vi "XYZ_XYStage_Status.vi"(4 "Model":string, 5 "error in (no error)":errorcluster, 7 "nStatusTries":i32=100, 8 "VISA resource name":refnum<visa-resource-name>="COM1") -> (0 "error out":errorcluster, 2 "Successs":bool, 3 "VISA resource name out":refnum<visa-resource-name>="COM1")   [LabVIEW 2013]
doc: "Sends STATUS command every 50 ms up to nStatusTries times.\nIf reply 'N' is received within nStatusTries times, then returns with Success = TRUE,\nelse returns with Success = FALSE."
uses:
  <vilib>/Instr/_visa.llb/VISA Configure Serial Port (Instr).vi
  Global.vi
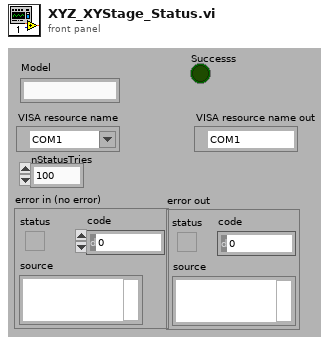
[diagram p1: front panel]
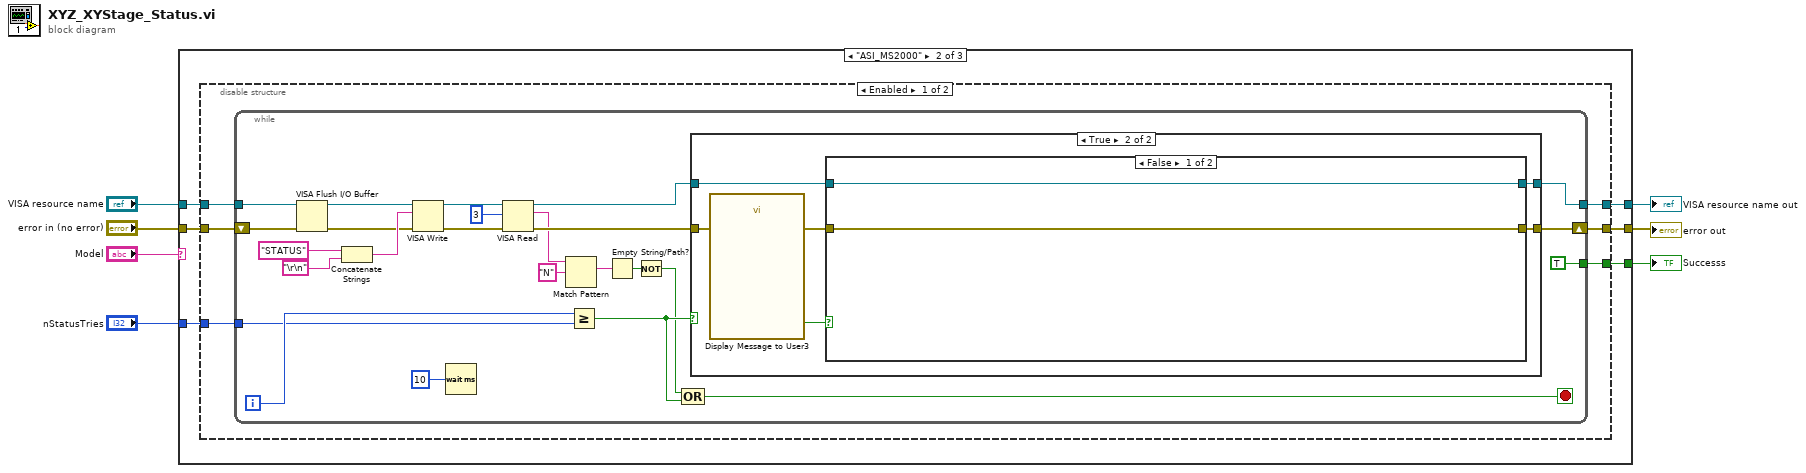
[diagram p0: block diagram]
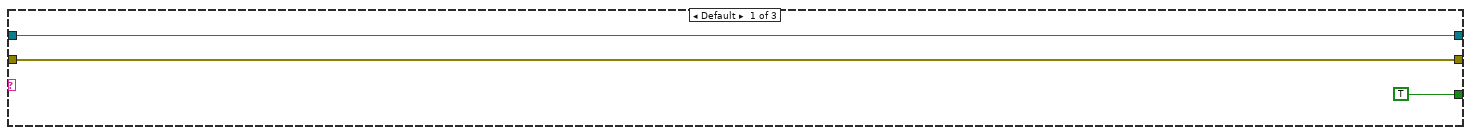
[diagram p2: hidden frame]
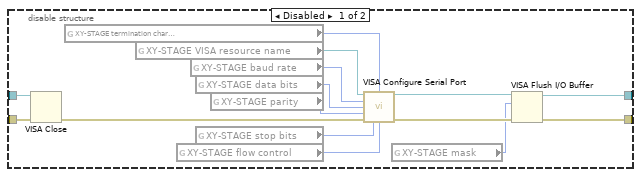
[diagram p5: hidden frame]
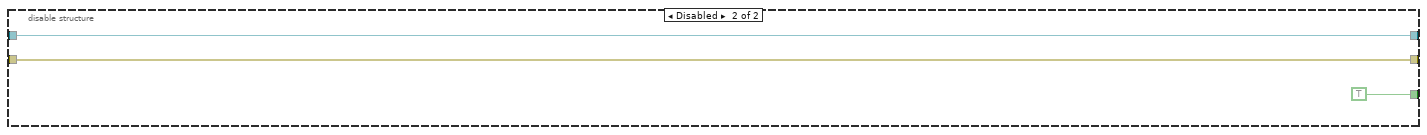
[diagram p6: hidden frame]
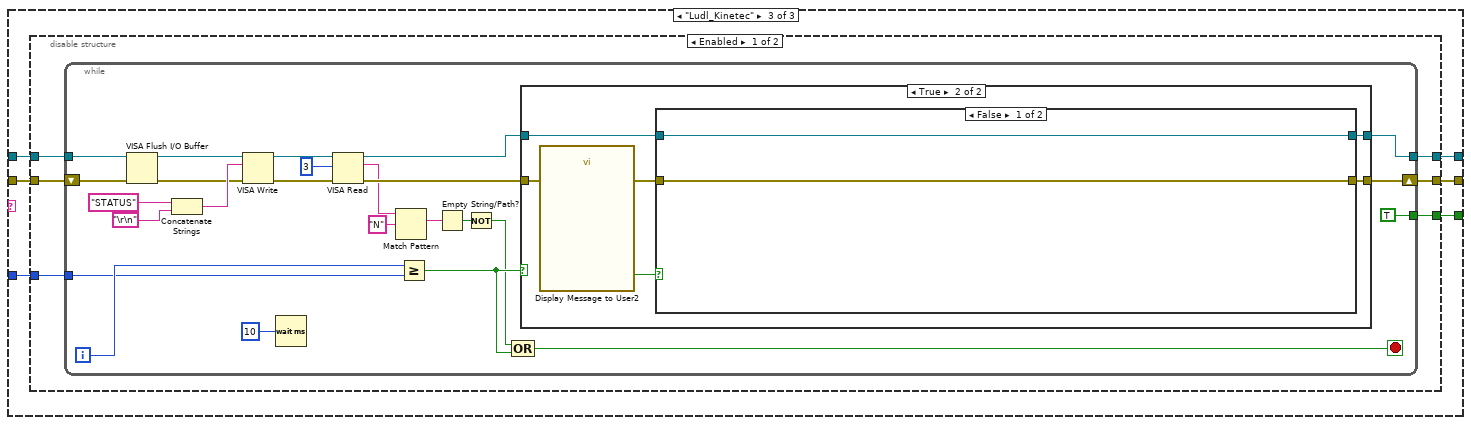
[diagram p7: hidden frame]
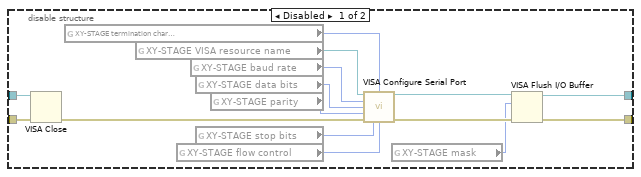
[diagram p10: hidden frame]
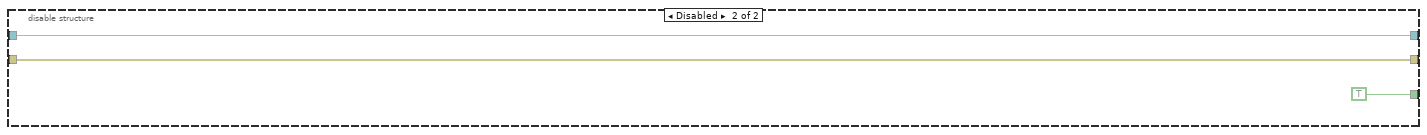
[diagram p11: hidden frame]
diagram:
  n1 = case shown="\"ASI_MS2000\"" "Model" {
    tunnel: [w9 w13 w84] -> w7
    tunnel: "error in (no error)" -> [w9 w16 w87]
    tunnel: "VISA resource name" -> [w8 w15 w86]
    tunnel: [TRUE w14 w85] -> w4
    tunnel: "nStatusTries" -> [_ w12 w83]
    tunnel: [w8 w11 w82] -> w1
    frame Default {
    }
    frame "ASI_MS2000" {
      n2 = disable-structure shown="Enabled" {
        disable-tunnel: w16 -> [w22 w81]
        disable-tunnel: w15 -> [w21 w79]
        disable-tunnel: [w20 TRUE] -> w14
        disable-tunnel: [w19 w81] -> w13
        disable-tunnel: w12 -> [w18 _]
        disable-tunnel: [w17 w79] -> w11
        frame Enabled {
          n3 = while {
            tunnel: w21 -> [w46]
            tunnel: [TRUE] -> w20
            shift-right: [w42] -> w19
            shift-left: w22 -> [w45]
            tunnel: w18 -> [w41]
            tunnel: [w28] -> w17
            i -> [w44]
            stop <- w47 stop-if-true
            n4 = VISA Flush I/O Buffer(VISA resource name=w46, error in (no error)=w45) -> (VISA resource name out=w33:refnum<visa-resource-name>, error out=w32:errorcluster)  [unwired: 1 in]
            n5 = Concatenate Strings("STATUS" ("string"), "\r\n") -> (w38:string)
            n6 = VISA Write(VISA resource name=w33, write buffer=w38, error in (no error)=w32) -> (VISA resource name out=w37:refnum<visa-resource-name>, error out=w35:errorcluster)  [unwired: 1 out]
            n7 = Wait (ms)(milliseconds to wait=u32 10) -> ()  [unwired: 1 out]
            n8 = VISA Read(VISA resource name=w37, byte count=u32 3, error in (no error)=w35) -> (VISA resource name out=w30:refnum<visa-resource-name>, read buffer=w25:string, error out=w29:errorcluster)  [unwired: 1 out]
            n9 = Match Pattern(string=w25, regular expression="N") -> (match substring=w27:string)  [unwired: 1 in, 3 out]
            n10 = Greater Or Equal?(x=w44, y=w41) -> (x >= y?=w31:bool)
            n11 = Empty String/Path?(string/path=w27) -> (empty?=w24:bool)
            n12 = Not(x=w24) -> (.not. x?=w23:bool)
            n13 = Compound Arithmetic op=OR(w23, w31) -> (w47:bool)
            n14 = case shown="True" w31 {
              tunnel: w30 -> [w48 w55]
              tunnel: w29 -> [w49 w53]
              tunnel: [w49 w51] -> w42
              tunnel: [w48 w50] -> w28
              frame False {
              }
              frame True {
                n15 = call "Display Message to User3"("error in (no error)"=w53) -> ("error out"=w52:errorcluster, "OK"=w54:bool)  [unwired: 9 in]
                n16 = case shown="False" w54 {
                  tunnel: w55 -> [w56 w61]
                  tunnel: w52 -> [w57 w60]
                  tunnel: [w57 w59] -> w51
                  tunnel: [w56 w58] -> w50
                  frame False {
                  }
                  frame True {
                    n17 = disable-structure shown="Enabled" {
                      disable-tunnel: w61 -> [w76 w77]
                      disable-tunnel: w60 -> [w75 w78]
                      disable-tunnel: [w63 w78] -> w59
                      disable-tunnel: [w62 w77] -> w58
                      frame Disabled {
                        n18 = VISA Close(VISA resource name=w76, error in (no error)=w75) -> (error out=w64:errorcluster)
                        n19 = global read "Global.vi" "XY-STAGE termination char\n(0xA = '\\n' = LF)"() -> (w72:u8)
                        n20 = global read "Global.vi" "XY-STAGE VISA resource name"() -> (w65:refnum<visa-resource-name>)
                        n21 = global read "Global.vi" "XY-STAGE flow control"() -> (w67:u16)
                        n22 = global read "Global.vi" "XY-STAGE baud rate"() -> (w69:u32)
                        n23 = global read "Global.vi" "XY-STAGE data bits"() -> (w70:u16)
                        n24 = global read "Global.vi" "XY-STAGE stop bits"() -> (w68:u16)
                        n25 = global read "Global.vi" "XY-STAGE parity"() -> (w71:enum16{"None", "Odd", "Even", "Mark", "Space"})
                        n26 = call-poly "VISA Configure Serial Port"("VISA resource name"=w65, "termination char\n(0xA = '\\n' = LF)"=w72, "baud rate (9600)"=w69, "data bits (8)"=w70, "parity (0:none)"=w71, "error in (no error)"=w64, "stop bits (10: 1 bit)"=w68, "flow control (0:none)"=w67) -> ("VISA resource name out"=w74:refnum<visa-resource-name>, "error out"=w73:errorcluster)  [unwired: 6 in]
                        n27 = global read "Global.vi" "XY-STAGE mask"() -> (w66:u16)
                        n28 = VISA Flush I/O Buffer(VISA resource name=w74, mask (16)=w66, error in (no error)=w73) -> (VISA resource name out=w62:refnum<visa-resource-name>, error out=w63:errorcluster)
                      }
                      frame Enabled {
                      }
                    }
                  }
                }
              }
            }
          }
        }
        frame Disabled {
        }
      }
    }
    frame "Ludl_Kinetec" {
      n29 = disable-structure shown="Enabled" {
        disable-tunnel: w87 -> [w93 w152]
        disable-tunnel: w86 -> [w92 w150]
        disable-tunnel: [w91 TRUE] -> w85
        disable-tunnel: [w90 w152] -> w84
        disable-tunnel: w83 -> [w89 _]
        disable-tunnel: [w88 w150] -> w82
        frame Enabled {
          n30 = while {
            tunnel: w92 -> [w117]
            tunnel: [TRUE] -> w91
            shift-right: [w113] -> w90
            shift-left: w93 -> [w116]
            tunnel: w89 -> [w112]
            tunnel: [w99] -> w88
            i -> [w115]
            stop <- w118 stop-if-true
            n31 = VISA Flush I/O Buffer(VISA resource name=w117, error in (no error)=w116) -> (VISA resource name out=w104:refnum<visa-resource-name>, error out=w103:errorcluster)  [unwired: 1 in]
            n32 = Concatenate Strings("STATUS" ("string"), "\r\n") -> (w109:string)
            n33 = VISA Write(VISA resource name=w104, write buffer=w109, error in (no error)=w103) -> (VISA resource name out=w108:refnum<visa-resource-name>, error out=w106:errorcluster)  [unwired: 1 out]
            n34 = Wait (ms)(milliseconds to wait=u32 10) -> ()  [unwired: 1 out]
            n35 = VISA Read(VISA resource name=w108, byte count=u32 3, error in (no error)=w106) -> (VISA resource name out=w101:refnum<visa-resource-name>, read buffer=w96:string, error out=w100:errorcluster)  [unwired: 1 out]
            n36 = Match Pattern(string=w96, regular expression="N") -> (match substring=w98:string)  [unwired: 1 in, 3 out]
            n37 = Greater Or Equal?(x=w115, y=w112) -> (x >= y?=w102:bool)
            n38 = Empty String/Path?(string/path=w98) -> (empty?=w95:bool)
            n39 = Not(x=w95) -> (.not. x?=w94:bool)
            n40 = Compound Arithmetic op=OR(w94, w102) -> (w118:bool)
            n41 = case shown="True" w102 {
              tunnel: w101 -> [w119 w126]
              tunnel: w100 -> [w120 w124]
              tunnel: [w120 w122] -> w113
              tunnel: [w119 w121] -> w99
              frame False {
              }
              frame True {
                n42 = call "Display Message to User2"("error in (no error)"=w124) -> ("error out"=w123:errorcluster, "OK"=w125:bool)  [unwired: 9 in]
                n43 = case shown="False" w125 {
                  tunnel: w126 -> [w127 w132]
                  tunnel: w123 -> [w128 w131]
                  tunnel: [w128 w130] -> w122
                  tunnel: [w127 w129] -> w121
                  frame False {
                  }
                  frame True {
                    n44 = disable-structure shown="Enabled" {
                      disable-tunnel: w132 -> [w147 w148]
                      disable-tunnel: w131 -> [w146 w149]
                      disable-tunnel: [w134 w149] -> w130
                      disable-tunnel: [w133 w148] -> w129
                      frame Disabled {
                        n45 = VISA Close(VISA resource name=w147, error in (no error)=w146) -> (error out=w135:errorcluster)
                        n46 = global read "Global.vi" "XY-STAGE termination char\n(0xA = '\\n' = LF)"() -> (w143:u8)
                        n47 = global read "Global.vi" "XY-STAGE VISA resource name"() -> (w136:refnum<visa-resource-name>)
                        n48 = global read "Global.vi" "XY-STAGE flow control"() -> (w138:u16)
                        n49 = global read "Global.vi" "XY-STAGE baud rate"() -> (w140:u32)
                        n50 = global read "Global.vi" "XY-STAGE data bits"() -> (w141:u16)
                        n51 = global read "Global.vi" "XY-STAGE stop bits"() -> (w139:u16)
                        n52 = global read "Global.vi" "XY-STAGE parity"() -> (w142:enum16{"None", "Odd", "Even", "Mark", "Space"})
                        n53 = call-poly "VISA Configure Serial Port"("VISA resource name"=w136, "termination char\n(0xA = '\\n' = LF)"=w143, "baud rate (9600)"=w140, "data bits (8)"=w141, "parity (0:none)"=w142, "error in (no error)"=w135, "stop bits (10: 1 bit)"=w139, "flow control (0:none)"=w138) -> ("VISA resource name out"=w145:refnum<visa-resource-name>, "error out"=w144:errorcluster)  [unwired: 6 in]
                        n54 = global read "Global.vi" "XY-STAGE mask"() -> (w137:u16)
                        n55 = VISA Flush I/O Buffer(VISA resource name=w145, mask (16)=w137, error in (no error)=w144) -> (VISA resource name out=w133:refnum<visa-resource-name>, error out=w134:errorcluster)
                      }
                      frame Enabled {
                      }
                    }
                  }
                }
              }
            }
          }
        }
        frame Disabled {
        }
      }
    }
  }
  "error out" <- w7
  "Successs" <- w4
  "VISA resource name out" <- w1
